vi "sv_Prepare Resample Data (DBL Array).vi"(11 "Array":dbl[][](array[numeric])) -> (0 "channel count":i32, 1 "signal len":i32, 3 "Y":dbl[](array[numeric]) format="%.2f")   [LabVIEW 2017, in "SoundVib_Resampling.lvlib"]
uses:
  <vilib>/addons/Sound and Vibration/Order Analysis/Resample Order Tracking/SoundVib_Resampling.lvlib
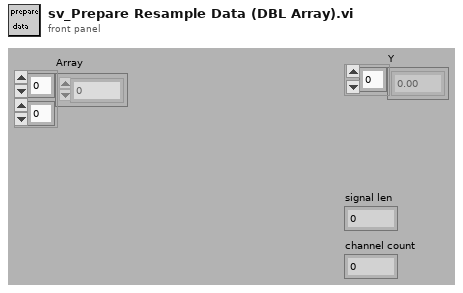
[diagram p1: front panel]
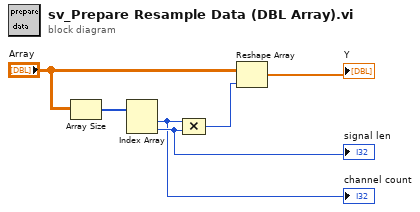
[diagram p0: block diagram]
diagram:
  n1 = Array Size(array="Array") -> (size(s)=w6:i32[])
  n2 = Index Array(array=w6) -> (element #1=w1:i32, element #2=w5:i32)  [unwired: 2 in]
  "channel count" <- w1
  "signal len" <- w5
  n3 = Compound Arithmetic op=MULTIPLY(w1, w5) -> (w3:i32)
  n4 = Reshape Array("Array", w3) -> (→"Y":dbl[])
